vi "Query_laser.vi"(6 "Reset?":bool, 7 "error in (no error)":errorcluster, 9 "String in":string="O?\n", 10 "VISA resource name":refnum<visa-resource-name>="COM8") -> (0 "error out":errorcluster, 1 "was busy?":bool, 2 "String out":string, 3 "VISA resource name 2":refnum<visa-resource-name>)   [LabVIEW 2011]
panel:
  in  "Busy":bool
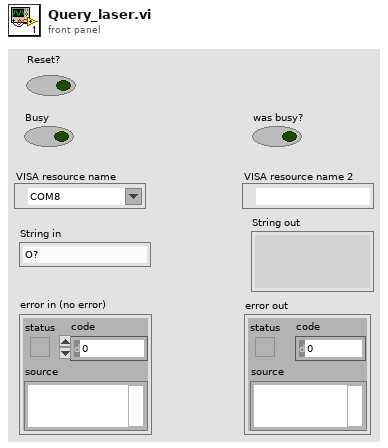
[diagram p1: front panel]
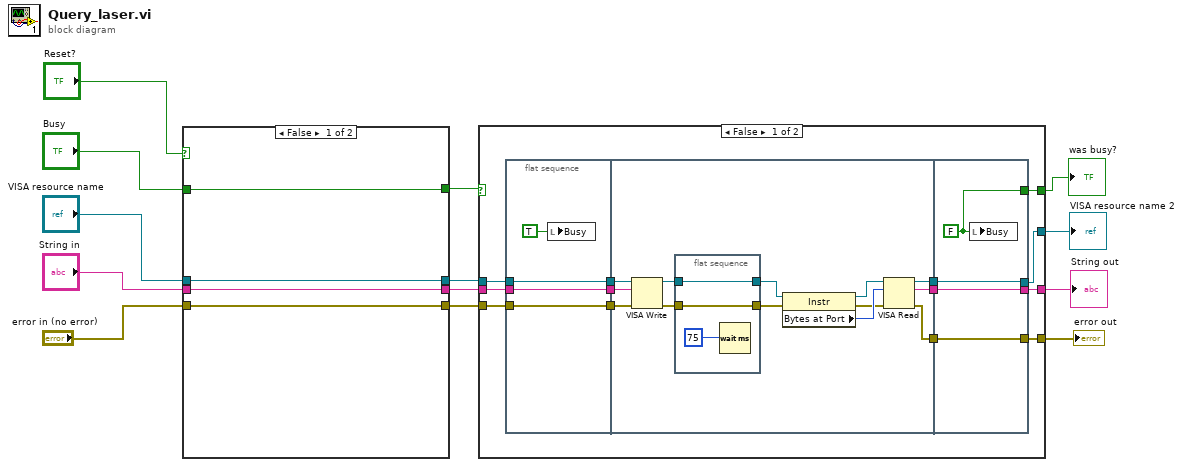
[diagram p0: block diagram]
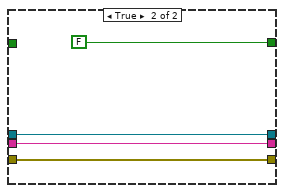
[diagram p2: hidden frame]
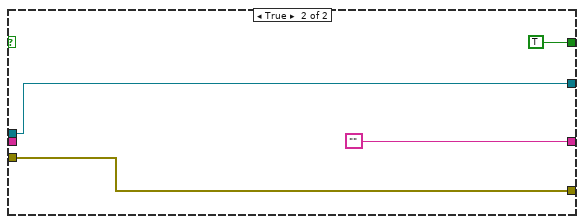
[diagram p3: hidden frame]
diagram:
  n1 = case shown="False" "Reset?" {
    tunnel: "Busy" -> [w17 _]
    tunnel: [w17 FALSE] -> w7
    tunnel: "error in (no error)" -> [w16 w18]
    tunnel: [w16 w18] -> w5
    tunnel: "String in" -> [w15 w19]
    tunnel: [w15 w19] -> w3
    tunnel: "VISA resource name" -> [w14 w20]
    tunnel: [w14 w20] -> w1
    frame False {
    }
    frame True {
    }
  }
  n2 = case shown="False" w7 {
    tunnel: w3 -> [w34 _]
    tunnel: [w33 ""] -> w13
    tunnel: [w32 w62] -> w12
    tunnel: w5 -> [w31 w62]
    tunnel: w1 -> [w30 w61]
    tunnel: [w23 w61] -> w11
    tunnel: [w22 TRUE] -> w10
    frame False {
      n3 = flat-sequence {
        tunnel: w30 -> [w36]
        tunnel: w31 -> [w37]
        tunnel: w34 -> [w38]
        tunnel: [w38] -> w29
        tunnel: [w37] -> w28
        tunnel: [w36] -> w27
        tunnel: w29 -> [w44]
        tunnel: w28 -> [w41]
        tunnel: w27 -> [w40]
        tunnel: [w43] -> w26
        tunnel: [w42] -> w25
        tunnel: [w39] -> w24
        tunnel: [w57] -> w32
        tunnel: [w58] -> w33
        tunnel: w26 -> [w58]
        tunnel: w25 -> [w57]
        tunnel: w24 -> [w56]
        tunnel: [w56] -> w23
        tunnel: [w55] -> w22
        frame #0 {
          n4 = local write "Busy"(TRUE) -> ()
        }
        frame #1 {
          n5 = VISA Write(VISA resource name=w40, write buffer=w44, error in (no error)=w41) -> (VISA resource name out=w45:refnum<visa-resource-name>, error out=w46:errorcluster)  [unwired: 1 out]
          n6 = flat-sequence {
            tunnel: w45 -> [w53]
            tunnel: [w53] -> w49
            tunnel: w46 -> [w52]
            tunnel: [w52] -> w47
            frame #0 {
              n7 = Wait (ms)(milliseconds to wait=75) -> ()  [unwired: 1 out]
            }
          }
          n8 = property class="Instr"(reference=w49, error in=w47) -> (reference out=w50:refnum<visa-resource-name>, error out=w48:errorcluster, "Bytes at Port"=w51:u32)
          n9 = VISA Read(VISA resource name=w50, byte count=w51, error in (no error)=w48) -> (VISA resource name out=w39:refnum<visa-resource-name>, read buffer=w43:string, error out=w42:errorcluster)  [unwired: 1 out]
        }
        frame #2 {
          w55 = FALSE
          n10 = local write "Busy"(w55) -> ()
        }
      }
    }
    frame True {
    }
  }
  "String out" <- w13
  "error out" <- w12
  "VISA resource name 2" <- w11
  "was busy?" <- w10
